vi "Channel Check.vi"(8 "error in (no error)":errorcluster, 10 "Channel":u16, 11 "BS120x in":refnum<class "BS120x.lvclass">) -> (0 "error out":errorcluster, 3 "BS120x out":refnum<class "BS120x.lvclass">)   [LabVIEW 2021, in "BS120x Driver.lvlib" / "BS120x.lvclass"]
uses:
  BS120x.lvclass
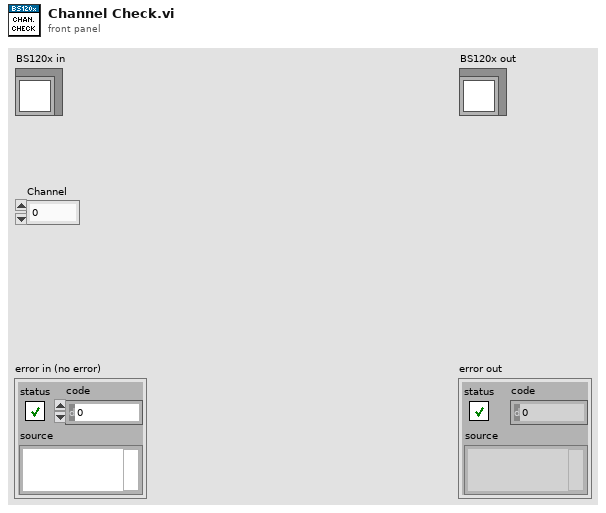
[diagram p1: front panel]
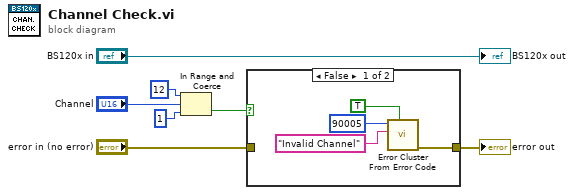
[diagram p0: block diagram]
diagram:
  n1 = In Range and Coerce(upper limit=u16 12, x="Channel", lower limit=u16 1) -> (In Range?=w6:bool)  [unwired: 1 out]
  n2 = case shown="False" w6 {
    tunnel: "error in (no error)" -> [_ w12]
    tunnel: [w8 w12] -> w1
    frame False {
      n3 = call <vilib>:"Error Cluster From Error Code.vi"("show call chain? (False)"=TRUE, "error message (\"\")"="Invalid Channel", "error code (0)"=90005) -> ("error out"=w8:errorcluster)  [unwired: 6 in]
    }
    frame True {
    }
  }
  "error out" <- w1
  "BS120x out" <- "BS120x in"
